vi "usbpt104+usbTC-arduino control PWM (concurrent6).vi"(10 "Mains Frequency":i16(ring) items=["50 Hz", "60 Hz"], 11 "Digital in":refnum<vi>) -> (2 "Handle 2":i16, 3 "Handle":i16)   [LabVIEW 2015]
uses:
  usbtc08.dll
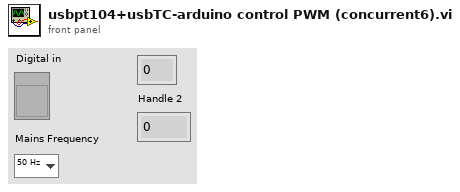
[diagram p1: front panel]
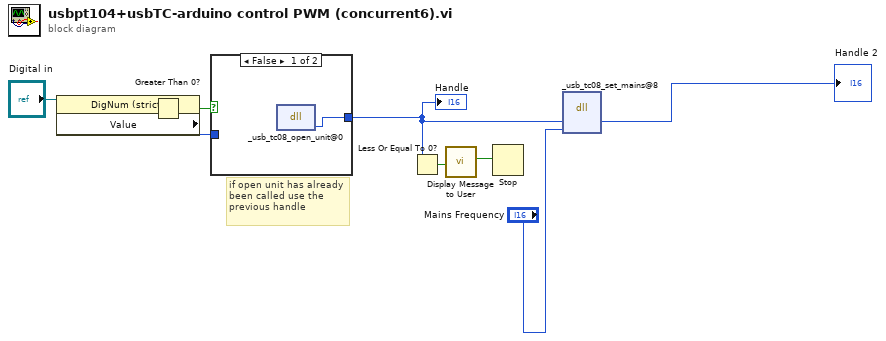
[diagram p0: block diagram]
diagram:
  # "if open unit has already been called use the previous handle"
  n1 = property class="DigNum (strict)"(reference="Digital in") -> ("Value"=w6:i16)  [unwired: 1 in, 2 out]
  n2 = Greater Than 0?(x=w6) -> (x > 0?=w7:bool)
  n3 = case shown="False" w7 {
    tunnel: [w9 w10] -> w5
    tunnel: w6 -> [_ w10]
    frame False {
      n4 = dll-call lib="usbtc08.dll" fn="_usb_tc08_open_unit@0" label="OpenUnit"() -> ("Handle"=w9:i16)  [unwired: 3 in, 2 out]
    }
    frame True {
    }
  }
  "Handle" <- w5
  n5 = Less Or Equal To 0?(x=w5) -> (x <= 0?=w4:bool)
  n6 = call "Display Message to User"("Enable"=w4) -> ("OK"=w3:bool)  [unwired: 9 in, 1 out]
  n7 = Stop(stop? (T)=w3) -> ()
  n8 = dll-call lib="usbtc08.dll" fn="_usb_tc08_set_mains@8" label="Set Mains"("Handle"=w5, "sixtyHertz"="Mains Frequency") -> ("Handle"=→"Handle 2":i16)  [unwired: 5 in, 2 out]
